vi "TEST - No of Elements in Cluster.vi"(8 "error in (no error)":errorcluster) -> (0 "error out":errorcluster, 2 "pass":bool)   [LabVIEW 2020, in "test_openg_variant.lvlib"]
uses:
  test_openg_variant.lvlib
  <userlib>/_OpenG.lib/error/error.llb/openg_error.lvlib
  source/library/openg_variant.lvlib
panel:
  out "Failures":T1(array[cluster])
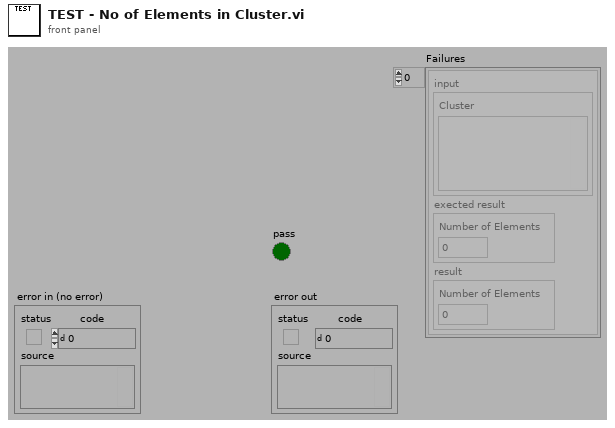
[diagram p1: front panel]
types:
  T1 = cluster{"input":cluster{"Cluster":variant}, "exected result":cluster{"Number of Elements":u16}, "result":cluster{"Number of Elements":u16}}[]
  T2 = cluster{"input":cluster{"Cluster":variant}, "exected result":cluster{"Number of Elements":u16}, "result":cluster{"Number of Elements":u16}}
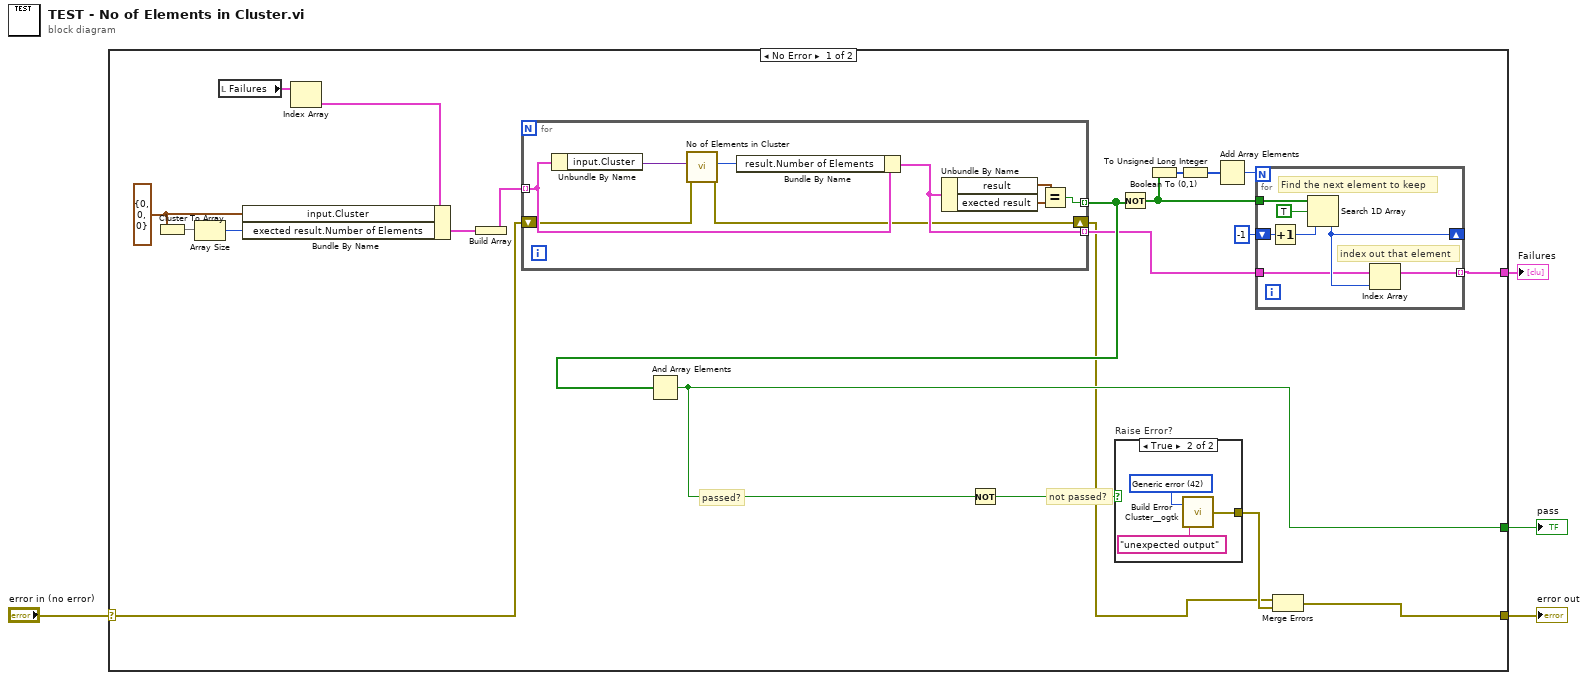
[diagram p0: block diagram]
diagram:
  n1 = case shown="No Error" "error in (no error)" {
    selector: "error in (no error)" -> [w11 w45]
    tunnel: [w22 _] -> w4
    tunnel: [w25 w45] -> w2
    tunnel: [w14 _] -> w1
    frame No Error {
      w7 = cluster{i32, i32, i32} {0, 0, 0}
      # "not passed?"
      # "passed?"
      n2 = Cluster To Array(cluster=w7) -> (array=w6:i32[])
      n3 = Array Size(array=w6) -> (size(s)=w5:i32)
      n4 = local read "Failures"() -> (w9:T1)
      n5 = Index Array(array=w9) -> (element=w8:T2)  [unwired: 1 in]
      n6 = Bundle By Name(cluster=w8, "input.Cluster"=w7, "exected result.Number of Elements"=w5) -> (w13:T2)
      n7 = Build Array(w13) -> (w12:T1)
      n8 = for {
        tunnel: w12 -> [w40] mode=indexing
        tunnel: [w41] -> w16 mode=indexing
        tunnel: [w39] -> w15 mode=indexing
        shift-right: [w35] -> w10
        shift-left: w11 -> [w34]
        n9 = Unbundle By Name(w40) -> ("input.Cluster"=w36:variant)
        n10 = call "No of Elements in Cluster.vi"("error in (no error)"=w34, "Cluster"=w36) -> ("error out"=w35:errorcluster, "Number of Elements"=w33:u16)  [unwired: 8 in]
        n11 = Bundle By Name(cluster=w40, "result.Number of Elements"=w33) -> (w39:T2)
        n12 = Unbundle By Name(w39) -> ("result"=w38:cluster{"Number of Elements":u16}, "exected result"=w37:cluster{"Number of Elements":u16})
        n13 = Equal?(x=w38, y=w37) -> (x = y?=w41:bool)
      }
      n14 = And Array Elements(Boolean array=w16) -> (logical AND=w22:bool)
      n15 = Not(x=w22) -> (.not. x?=w23:bool)
      n16 = case "Raise Error?" shown="True" w23 {
        tunnel: [_ w42] -> w24
        frame False {
        }
        frame True {
          w43 = 42 items=["No error", "Argument error", "Memory is full", "Out of zone", "End of file", "File already open", "Generic file I/O error", "File not found", "File permission error", "Disk is full", "Duplicate path", "Too many files open", "System feature not enabled", "Resource file not found", "Cannot add resource", "Resource not found", "Image not found", "Image memory error", "Pen does not exist", "Config type invalid", "Config token not found", "Config parse error", "Config memory error", "Bad external code format", "Bad external code offset", "External code not present", "Null window", "Destroy window error", "Null menu", "Print aborted", "Bad print record", "Print driver error", "Windows error during printing", "Memory error during printing", "Print dialog error", "Generic print error", "Invalid device refnum", "Device not found", "Device parameter error", "Device unit error", "Cannot open device", "Device call aborted", "Generic error", "Cancelled by user", "Object ID too low", "Object ID too high", "Object not in heap", "Unknown heap", "Unknown object (invalid DefProc)", "Unknown object (DefProc not in table)", "Message out of range", "Invalid (null) method", "Unknown message", "Manager call not supported", "Bad address", "Network operation in progress", "Network operation timed out", "Connection is busy", "Network attribute not supported", "Network error", "Address in use", "System out of memory", "Connection aborted", "Connection refused", "Not connected", "Already connected", "Connection closed", "Initialization error (interapplication manager)", "Bad occurrence", "Wait on unbound occurrence handler", "Occurrence queue overflow", "Datalog type conflict", "Unused", "Unrecognized type (interapplication manager)", "Memory corrupt", "Failed to make temporary DLL", "Old CIN version", "Drag socket not found", "Failed to load drop-object", "Failed to register OLE object", "Failed to release OLE object", "Format specifier type mismatch", "Unknown format specifier", "Too few format specifiers", "Too many format specifiers", "Scan failed", "Newer CIN version", "Error converting to variant", "Runtime menu error", "Password tampered", "Variant attribute not found", "Incompatible variant data type", "Event data is not available", "Event Store is not present", "Occurrence is not found", "Event Queue is not created", "Event info is not available", "Refnum passed is NULL", "Error retrieving Class GUID", "Error retrieving CoClass GUID", "Error retrieving TypeLib GUID.", "Bad built application magic bytes.", "Specific driver is different from the specific driver associated with the Logical Name.", "There is no session opened to the class driver.", "Max Error", "MAX - Error with config objects", "MAX - Error loading configuration", "MAX - Group not supported"]
          n17 = call <userlib>:"Build Error Cluster__ogtk.vi"("String to Prepend to source (\"\")"="unexpected output" ("String to Prepend to source (\"\")"), "code"=w43) -> ("error out"=w42:errorcluster)
        }
      }
      n18 = Not(x=w16) -> (.not. x?=w18:bool[])
      n19 = Boolean To (0,1)(Boolean=w18) -> (0, 1=w19:i16[])
      n20 = To Unsigned Long Integer(number=w19) -> (unsigned 32bit integer=w17:u32[])
      n21 = Add Array Elements(numeric array=w17) -> (sum=w20:u32)
      n22 = for {
        N: w20 -> [_]
        tunnel: w15 -> [w28]
        tunnel: w18 -> [w32]
        shift-right: [w29] -> _
        shift-left: -1 ("start index (0)") -> [w30]
        tunnel: [w27] -> w14 mode=indexing
        # "index out that element"
        # "Find the next element to keep"
        n23 = Increment(x=w30) -> (x+1=w26:i32)
        n24 = Search 1D Array(1D array=w32, element=TRUE, start index (0)=w26) -> (index of element=w29:i32)
        n25 = Index Array(array=w28, index=w29) -> (element=w27:T2)
      }
      n26 = Merge Errors(w10, w24) -> (w25:errorcluster)
    }
    frame Error {
    }
  }
  "pass" <- w4
  "error out" <- w2
  "Failures" <- w1
